vi "Index Array (JSON).vi"(8 "error in":errorcluster, 9 "index":i32, 10 "JSON Array in":refnum<class "JSON Value.lvclass">) -> (0 "error out":errorcluster, 1 "JSON out":refnum<class "JSON Value.lvclass">)   [LabVIEW 2016, in "JSON Value.lvclass"]
doc: "Returns the JSON element of the JSON array at index."
uses:
  JSON Helper/JSON Value.lvclass
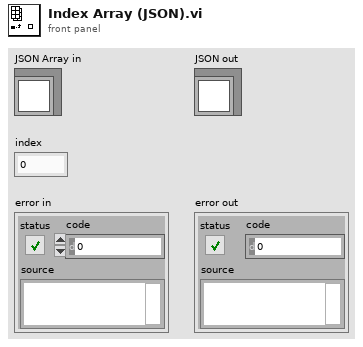
[diagram p1: front panel]
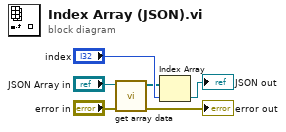
[diagram p0: block diagram]
diagram:
  n1 = call "get array data.vi"("error in (no error)"="error in", "JSON Helper in"="JSON Array in") -> ("error out"=→"error out":errorcluster, "JSON Array out"=w3:refnum<class "JSON Value.lvclass">[])  [unwired: 8 in]
  n2 = Index Array(array=w3, index="index") -> (element=→"JSON out":refnum<class "JSON Value.lvclass">)
